vi "Flags to Bit Mask.vi"(1 "Flags":T1) -> (0 "Bit Mask":u32)   [LabVIEW 2018, in "Toolkit.lvlib" / "SFTP File.lvclass"]
uses:
  SFTP File.lvclass
  API/Typedefs/Flags.ctl
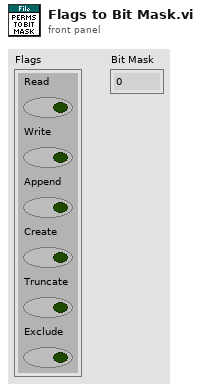
[diagram p1: front panel]
types:
  T1 = typedef "Toolkit.lvlib/SFTP File.lvclass/Flags.ctl" = cluster{"Read":bool, "Write":bool, "Append":bool, "Create":bool, "Truncate":bool, "Exclude":bool}
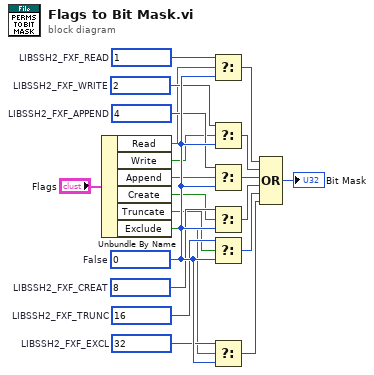
[diagram p0: block diagram]
diagram:
  w15 = u32 32  # LIBSSH2_FXF_EXCL
  w16 = u32 16  # LIBSSH2_FXF_TRUNC
  w17 = u32 8  # LIBSSH2_FXF_CREAT
  w18 = u32 4  # LIBSSH2_FXF_APPEND
  w19 = u32 2  # LIBSSH2_FXF_WRITE
  w20 = u32 1  # LIBSSH2_FXF_READ
  w21 = u32 0  # False
  n1 = Unbundle By Name("Flags") -> ("Read"=w13:bool, "Write"=w12:bool, "Append"=w11:bool, "Create"=w10:bool, "Truncate"=w9:bool, "Exclude"=w8:bool)
  n2 = Select(t=w20, s=w13, f=w21) -> (s? t:f=w7:u32)
  n3 = Select(t=w19, s=w12, f=w21) -> (s? t:f=w6:u32)
  n4 = Select(t=w18, s=w11, f=w21) -> (s? t:f=w5:u32)
  n5 = Select(t=w17, s=w10, f=w21) -> (s? t:f=w4:u32)
  n6 = Select(t=w16, s=w9, f=w21) -> (s? t:f=w3:u32)
  n7 = Select(t=w15, s=w8, f=w21) -> (s? t:f=w2:u32)
  n8 = Compound Arithmetic op=OR(w7, w6, w5, w4, w3, w2) -> (→"Bit Mask":u32)
